vi "test Passes If Timestamps Are Equal Within 1 Minute Delta.vi"(8 "error in (no error)":errorcluster, 11 "TestCase in":refnum<class "Pass If Equal Timestamp Test Case.lvclass">) -> (0 "error out":errorcluster, 3 "TestCase out":refnum<class "Pass If Equal Timestamp Test Case.lvclass">)   [LabVIEW 2015, in "Pass If Equal Timestamp Test Case.lvclass"]
uses:
  Pass If Equal Timestamp Test Case.lvclass
  <vilib>/addons/_JKI Toolkits/VI Tester/TestCase.llb/TestCase.lvclass
  VITAC.lvlib
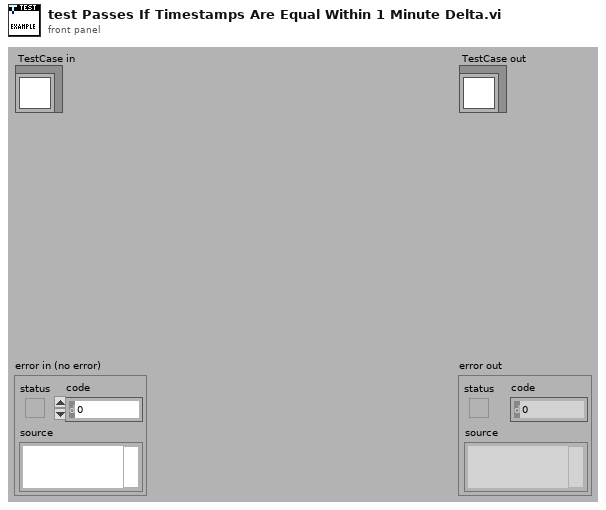
[diagram p1: front panel]
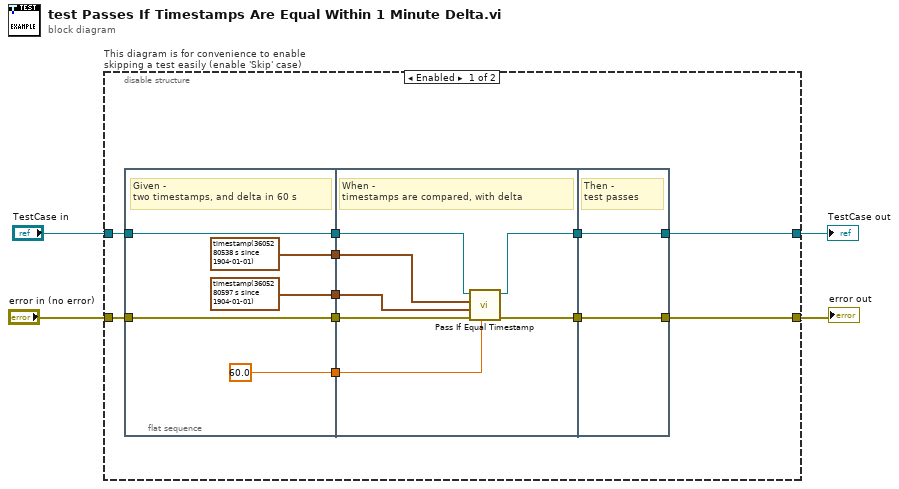
[diagram p0: block diagram]
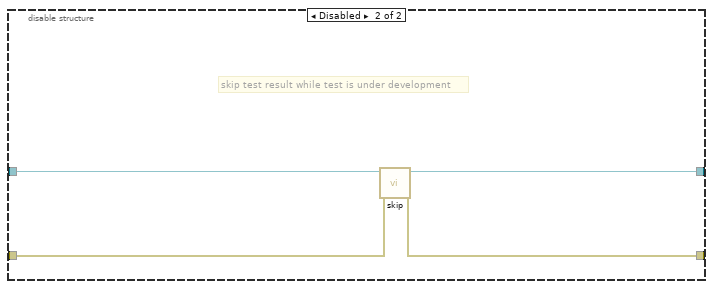
[diagram p2: hidden frame]
diagram:
  n1 = disable-structure "This diagram is for convenience to enable skipping a test easily (enable 'Skip' case)" shown="Enabled" {
    disable-tunnel: "TestCase in" -> [w10 w33]
    disable-tunnel: [w13 w31] -> w1
    disable-tunnel: [w12 w32] -> w3
    disable-tunnel: "error in (no error)" -> [w11 w30]
    frame Enabled {
      n2 = flat-sequence {
        tunnel: w11 -> [w19]
        tunnel: w10 -> [w20]
        tunnel: [w20] -> w9
        tunnel: [w19] -> w8
        tunnel: [timestamp(3605280538.17 s since 1904-01-01)] -> w7
        tunnel: [timestamp(3605280597.1703305 s since 1904-01-01) ("Time Stamp")] -> w6
        tunnel: [60.0] -> w5
        tunnel: [w26] -> w15
        tunnel: w9 -> [w27]
        tunnel: w8 -> [w24]
        tunnel: [w25] -> w14
        tunnel: w7 -> [w23]
        tunnel: w6 -> [w22]
        tunnel: w5 -> [w21]
        tunnel: [w29] -> w12
        tunnel: w15 -> [w28]
        tunnel: w14 -> [w29]
        tunnel: [w28] -> w13
        frame #0 {
          # "Given - \ntwo timestamps, and delta in 60 s"
        }
        frame #1 {
          # "When - \ntimestamps are compared, with delta"
          n3 = call "Pass If Equal Timestamp.vi"("delta (optional)"=w21, "error in (no error)"=w24, "actual timestamp"=w22, "expected timestamp"=w23, "TestCase in"=w27) -> ("error out"=w25:errorcluster, "TestCase out"=w26:refnum<class "Pass If Equal Timestamp Test Case.lvclass">)  [unwired: 5 in]
        }
        frame #2 {
          # "Then - \ntest passes"
        }
      }
    }
    frame Disabled {
      # "skip test result while test is under development"
      n4 = call <vilib>:"skip.vi"("error in (no error)"=w30, "TestCase in"=w33) -> ("error out"=w32:errorcluster, "TestCase out"=w31:refnum<class "Pass If Equal Timestamp Test Case.lvclass">)  [unwired: 8 in]
    }
  }
  "error out" <- w3
  "TestCase out" <- w1
